vi "poly_remove_nans_DBL.vi"(10 "input":dbl[](array[numeric]) format="%#_13g") -> (1 "indices":i32[](array[numeric]), 2 "output":dbl[](array[numeric]))   [LabVIEW 2015]
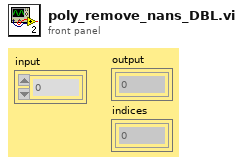
[diagram p1: front panel]
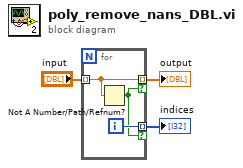
[diagram p0: block diagram]
diagram:
  n1 = for {
    tunnel: "input" -> [w6] mode=indexing
    tunnel: [w6] -> w2 mode=indexing if=w4
    tunnel: [w5] -> w1 mode=indexing if=w4
    i -> [w5]
    n2 = Not A Number/Path/Refnum?(number/path/refnum=w6) -> (NaN/Path/Refnum?=w4:bool)
  }
  "output" <- w2
  "indices" <- w1
